vi "UHR-Fleezers Control (host) - 12.0.vi"() -> ()   [LabVIEW 2012] (continued)
            n680 = call "move to saved stage position.vi"("error in"=w1089, "Stage VISA resource name in"=w1090, "Position"="Stage Position To Establish FB", "Saved Stage Positions"=w1092) -> ("error out"=w1088:errorcluster)  [unwired: 1 out]
            n681 = local write "Stage Control Serial Error"(w1088) -> ()
          }
          frame #2 {
            n682 = call <vilib>:"Beep.vi"() -> ()  [unwired: 3 in, 9 out]
            n683 = Multiply(x="Wait (s)", y=u32 1000 ("milliseconds to wait")) -> (x*y=w1099:u32)
            n684 = property on="Trap Delta (MHz)" class="DigNum (strict)"("Val(Sgnl)"="Starting \nTrap Delta (MHz)") -> ()  [unwired: 2 in, 2 out]
            n685 = local write "Stage Moving"(FALSE ("Stage Moving")) -> ()
            n686 = Wait (ms)(milliseconds to wait=w1099) -> ()  [unwired: 1 out]
            n687 = property on="Tab Control 2" class="TabCtl (strict)"("Val(Sgnl)"=T6."Feedback on Trap Position" ("Value (Signaling)")) -> ()  [unwired: 2 in, 2 out]
            n688 = property on="Tab Control" class="TabCtl (strict)"("Val(Sgnl)"=T4."Trap Control (RF)" ("Value (Signaling)")) -> ()  [unwired: 2 in, 2 out]
          }
          frame #3 {
            n689 = property on="Set Reading to\nSetpoint" class="Bool (strict)"("Val(Sgnl)"=TRUE ("Value (Signaling)")) -> ()  [unwired: 2 in, 2 out]
            n690 = Wait (ms)(milliseconds to wait=u32 500) -> ()  [unwired: 1 out]
          }
          frame #4 {
            n691 = property on="Trap Pos. FB ON" class="Bool (strict)"("Val(Sgnl)"=TRUE ("Value (Signaling)")) -> ()  [unwired: 2 in, 2 out]
            n692 = Wait (ms)(milliseconds to wait=u32 250) -> ()  [unwired: 1 out]
          }
          frame #5 {
            n693 = case shown="False" "Trap Trig Fl." {
              frame False {
                n694 = case shown="True" "Green ON after FB ON?" {
                  selector: "Green ON after FB ON?" -> [_ w1114]
                  frame False {
                  }
                  frame True {
                    n695 = property on="Green Laser ON/Interlacing" class="Bool (strict)"("Val(Sgnl)"=w1114) -> ()  [unwired: 2 in, 2 out]
                  }
                }
              }
              frame True {
              }
            }
            n696 = case shown="True" "Remove Action Offset" {
              tunnel: TRUE ("Value (Signaling)") -> [w1111 w1112]
              frame False {
                n697 = property on="Remove Unwinding Offset" class="Bool (strict)"("Val(Sgnl)"=w1111) -> ()  [unwired: 2 in, 2 out]
              }
              frame True {
                n698 = property on="Remove Action Offset" class="Bool (strict)"("Val(Sgnl)"=w1112) -> ()  [unwired: 2 in, 2 out]
              }
            }
            n699 = Wait (ms)(milliseconds to wait=u32 250) -> ()  [unwired: 1 out]
          }
          frame #6 {
            n700 = property on="Start Saving" class="Bool (strict)"("Val(Sgnl)"=TRUE ("Value (Signaling)")) -> ()  [unwired: 2 in, 2 out]
            n701 = Wait (ms)(milliseconds to wait=u32 5000) -> ()  [unwired: 1 out]
          }
          frame #7 {
            w1118 = TRUE ("Value (Signaling)")
            n702 = property on="Rem fb disp offset" class="Bool (strict)"("Val(Sgnl)"=w1118) -> ()  [unwired: 2 in, 2 out]
            n703 = property on="Remove Offset" class="Bool (strict)"("Val(Sgnl)"=w1118) -> ()  [unwired: 2 in, 2 out]
            n704 = Wait (ms)(milliseconds to wait=u32 100) -> ()  [unwired: 1 out]
          }
          frame #8 {
            n705 = case shown="True" w1121 {
              frame False {
              }
              frame True {
                n706 = local write "Trap Trig. Fl."(TRUE ("Value (Signaling)")) -> ()
              }
            }
          }
          frame #9 {
            n707 = case shown="True" "Start dipping after?" {
              frame False {
              }
              frame True {
                n708 = flat-sequence {
                  frame #0 {
                    n709 = Multiply(x="Delay before dipping (s)", y=1000.0) -> (x*y=w1125:dbl)
                    n710 = Wait (ms)(milliseconds to wait=w1125) -> ()  [unwired: 1 out]
                  }
                  frame #1 {
                    n711 = property on="Dip for Protein" class="Bool (strict)"("Val(Sgnl)"=TRUE ("Value (Signaling)")) -> ()  [unwired: 2 in, 2 out]
                    n712 = local write "Scripts"(T1."Dipping" ("Scripts")) -> ()
                  }
                }
              }
            }
          }
        }
      }
      event "Fixed Traps Data\nScript": Value Change {
        n713 = event-data() -> ()  [unwired: 1 in, 5 out]
        n714 = flat-sequence {
          frame #0 {
            n715 = case shown="True" "Green ON" {
              frame False {
              }
              frame True {
                n716 = property on="Green Laser ON/Interlacing" class="Bool (strict)"("Val(Sgnl)"=TRUE) -> ()  [unwired: 2 in, 2 out]
              }
            }
            n717 = local write "Offset (nm)"(0.0 ("Offset (nm)")) -> ()
            n718 = property on="Sample Channel\nFlow" class="Bool (strict)"("Val(Sgnl)"=FALSE ("Value (Signaling)")) -> ()  [unwired: 2 in, 2 out]
            n719 = property on="Trap Delta (MHz)" class="DigNum (strict)"("Val(Sgnl)"="Fixed Traps Trap Delta (MHz)") -> ()  [unwired: 2 in, 2 out]
          }
          frame #1 {
            n720 = Wait (ms)(milliseconds to wait=u32 1000) -> ()  [unwired: 1 out]
          }
          frame #2 {
            n721 = local write "Start Saving"(TRUE ("Start Saving")) -> ()
          }
          frame #3 {
            n722 = local read "Bead Sep. Int. Time (s)"() -> (w1136:dbl)
            n723 = Multiply(x=w1136, y=1000.0) -> (x*y=w1138:dbl)
            n724 = Wait (ms)(milliseconds to wait=w1138) -> ()  [unwired: 1 out]
          }
          frame #4 {
            n725 = property on="Remove Offset" class="Bool (strict)"("Val(Sgnl)"=TRUE ("Value (Signaling)")) -> ()  [unwired: 2 in, 2 out]
          }
          frame #5 {
            n726 = property on="Dip for Protein" class="Bool (strict)"("Val(Sgnl)"="Start dipping after?") -> ()  [unwired: 2 in, 2 out]
          }
        }
      }
      event "Got DNA bead": Value Change {
        n727 = event-data() -> ()  [unwired: 1 in, 5 out]
        n728 = flat-sequence {
          frame #0 {
            n729 = local read "Daq spot flow on"() -> (w1143:bool)
            n730 = case shown="True" w1143 {
              frame False {
              }
              frame True {
                n731 = property on="Sample Channel\nFlow" class="Bool (strict)"("Val(Sgnl)"=TRUE ("Value (Signaling)")) -> ()  [unwired: 2 in, 2 out]
              }
            }
            n732 = property on="Got DNA bead" class="Bool"("Key Focus"=FALSE) -> ()  [unwired: 2 in, 2 out]
          }
          frame #1 {
            n733 = property on="Inject Pump 1" class="Bool (strict)"("Val(Sgnl)"=FALSE ("Value (Signaling)")) -> ()  [unwired: 2 in, 2 out]
          }
          frame #2 {
            n734 = property on="Cal/Data Acq. Spot" class="Bool (strict)"("Val(Sgnl)"=TRUE ("Value (Signaling)")) -> ()  [unwired: 2 in, 2 out]
          }
        }
      }
      event "Take Stepping Data": Value Change {
        n735 = event-data() -> ()  [unwired: 1 in, 5 out]
        n736 = local read "Save ave N"() -> (w1155:dbl)
        n737 = flat-sequence {
          tunnel: w1155 -> [w1157]
          tunnel: [w1157] -> w1150
          tunnel: [w1159] -> w1151
          tunnel: w1150 -> [w1159]
          tunnel: [w1161] -> w1152
          tunnel: w1151 -> [w1161]
          tunnel: [w1164] -> w1153
          tunnel: w1152 -> [w1164]
          tunnel: [w1166] -> w1154
          tunnel: w1153 -> [w1166]
          tunnel: [w1168] -> w1148
          tunnel: w1154 -> [w1168]
          tunnel: w1148 -> [w1171]
          tunnel: [w1171] -> w1147
          tunnel: w1147 -> [w1172]
          tunnel: [w1172] -> w1149
          tunnel: w1149 -> [w1178]
          frame #0 {
            n738 = property on="Save ave N" class="DigNum (strict)"("Val(Sgnl)"="Save ave factor") -> ()  [unwired: 2 in, 2 out]
          }
          frame #1 {
            n739 = Wait (ms)(milliseconds to wait=u32 100) -> ()  [unwired: 1 out]
          }
          frame #2 {
            n740 = local read "Offset 2 Start (MHz)"() -> (w1163:dbl)
            n741 = property on="Saved AOD Raster Scan Parameter Sets" class="Arr (strict)"("Index Values"=u32[] [2]) -> ()  [unwired: 2 in, 2 out]
            n742 = property on="Trap Delta (MHz)" class="DigNum (strict)"("Val(Sgnl)"=w1163) -> ()  [unwired: 2 in, 2 out]
          }
          frame #3 {
            n743 = property on="Load parameters" class="Bool (strict)"("Val(Sgnl)"=TRUE ("Value (Signaling)")) -> ()  [unwired: 2 in, 2 out]
          }
          frame #4 {
            n744 = Wait (ms)(milliseconds to wait=u32 100) -> ()  [unwired: 1 out]
          }
          frame #5 {
            n745 = property on="Trap Raster Scan" class="Bool (strict)"("Val(Sgnl)"=TRUE ("Value (Signaling)")) -> ()  [unwired: 2 in, 2 out]
          }
          frame #6 {
            n746 = Wait (ms)(milliseconds to wait=u32 1000) -> ()  [unwired: 1 out]
          }
          frame #7 {
            n747 = while {
              stop <- w1175 stop-if-true
              n748 = local read "Raster Scanning..."() -> (w1177:bool)
              n749 = local read "Saving..."() -> (w1176:bool)
              n750 = Not(x=w1176) -> (.not. x?=w1173:bool)
              n751 = Not(x=w1177) -> (.not. x?=w1174:bool)
              n752 = And(x=w1174, y=w1173) -> (x .and. y?=w1175:bool)
            }
          }
          frame #8 {
            n753 = property on="Save ave N" class="DigNum (strict)"("Val(Sgnl)"=w1178) -> ()  [unwired: 2 in, 2 out]
          }
        }
      }
      event "Step Size (nm)": Value Change {
        n754 = event-data() -> ()  [unwired: 1 in, 5 out]
        n755 = flat-sequence {
          frame #0 {
            n756 = property on="Saved AOD Raster Scan Parameter Sets" class="Arr (strict)"("Index Values"=u32[] [1]) -> ()  [unwired: 2 in, 2 out]
          }
          frame #1 {
            n757 = Multiply(x="N Steps", y="Step Size (nm)") -> (x*y=w1180:dbl)
            n758 = property on="Scan Speed AOD (nm/s) 2" class="DigNum (strict)"("Value"="Step Size (nm)") -> ()  [unwired: 2 in, 2 out]
            n759 = property on="Step Size AOD (nm) 2" class="DigNum (strict)"("Value"="Step Size (nm)") -> ()  [unwired: 2 in, 2 out]
            n760 = property on="Scan Range AOD (nm) 2" class="DigNum (strict)"("Value"=w1180) -> ()  [unwired: 2 in, 2 out]
          }
        }
      }
      event "Take Detection Laser\nImage": Value Change {
        n761 = event-data() -> ()  [unwired: 1 in, 5 out]
        n762 = flat-sequence {
          tunnel: [w1208] -> w1198
          tunnel: [w1207] -> w1191
          tunnel: [w1206] -> w1183
          tunnel: [w1211] -> w1199
          tunnel: w1198 -> [w1211]
          tunnel: [w1210] -> w1192
          tunnel: w1191 -> [w1210]
          tunnel: [w1209] -> w1184
          tunnel: w1183 -> [w1209]
          tunnel: [w1215] -> w1200
          tunnel: w1199 -> [w1215]
          tunnel: [w1214] -> w1193
          tunnel: w1192 -> [w1214]
          tunnel: [w1213] -> w1185
          tunnel: w1184 -> [w1213]
          tunnel: [w1221] -> w1201
          tunnel: w1200 -> [w1221]
          tunnel: [w1220] -> w1194
          tunnel: w1193 -> [w1220]
          tunnel: [w1219] -> w1186
          tunnel: w1185 -> [w1219]
          tunnel: [w1225] -> w1202
          tunnel: w1201 -> [w1225]
          tunnel: [w1224] -> w1195
          tunnel: w1194 -> [w1224]
          tunnel: [w1223] -> w1187
          tunnel: w1186 -> [w1223]
          tunnel: [w1229] -> w1203
          tunnel: w1202 -> [w1229]
          tunnel: [w1228] -> w1196
          tunnel: w1195 -> [w1228]
          tunnel: [w1227] -> w1188
          tunnel: w1187 -> [w1227]
          tunnel: [w1233] -> w1204
          tunnel: w1203 -> [w1233]
          tunnel: [w1232] -> w1197
          tunnel: w1196 -> [w1232]
          tunnel: [w1231] -> w1189
          tunnel: w1188 -> [w1231]
          tunnel: w1204 -> [w1239]
          tunnel: w1197 -> [w1238]
          tunnel: [w1236] -> w1190
          tunnel: w1189 -> [w1236]
          tunnel: w1190 -> [w1240]
          frame #0 {
            n763 = local read "Green Laser ON/Interlacing"() -> (w1208:bool)
            n764 = local read "Green laser mode"() -> (w1207:enum32{"Laser ON", "Laser OFF", "Interlace"})
            n765 = local read "Green FB On/Off"() -> (w1206:bool)
          }
          frame #1 {
            n766 = property on="Green FB On/Off" class="Bool (strict)"("Val(Sgnl)"=FALSE ("Value (Signaling)")) -> ()  [unwired: 2 in, 2 out]
          }
          frame #2 {
            n767 = property on="Green Laser ON/Interlacing" class="Bool (strict)"("Val(Sgnl)"=TRUE ("Value (Signaling)")) -> ()  [unwired: 2 in, 2 out]
            n768 = property on="Flip Green Filter" class="Bool (strict)"("Val(Sgnl)"=TRUE ("Value (Signaling)")) -> ()  [unwired: 2 in, 2 out]
            n769 = property on="Green laser mode" class="RadioBtnsControl (strict)"("Val(Sgnl)"=enum32{"Laser ON", "Laser OFF", "Interlace"}."Laser ON" ("Value (Signaling)")) -> ()  [unwired: 2 in, 2 out]
          }
          frame #3 {
            n770 = Wait (ms)(milliseconds to wait=u32 500) -> ()  [unwired: 1 out]
          }
          frame #4 {
            n771 = property on="Confocal Image" class="Bool (strict)"("Val(Sgnl)"=TRUE ("Value (Signaling)")) -> ()  [unwired: 2 in, 2 out]
          }
          frame #5 {
            n772 = Wait (ms)(milliseconds to wait=u32 2000) -> ()  [unwired: 1 out]
          }
          frame #6 {
            n773 = while {
              stop <- w1234 stop-if-true
              n774 = local read "Saving..."() -> (w1235:bool)
              n775 = Not(x=w1235) -> (.not. x?=w1234:bool)
            }
          }
          frame #7 {
            n776 = property on="Flip Green Filter" class="Bool (strict)"("Val(Sgnl)"=TRUE ("Value (Signaling)")) -> ()  [unwired: 2 in, 2 out]
            n777 = property on="Green Laser ON/Interlacing" class="Bool (strict)"("Val(Sgnl)"=w1239) -> ()  [unwired: 2 in, 2 out]
            n778 = property on="Green laser mode" class="RadioBtnsControl (strict)"("Val(Sgnl)"=w1238) -> ()  [unwired: 2 in, 2 out]
          }
          frame #8 {
            n779 = property on="Green FB On/Off" class="Bool (strict)"("Val(Sgnl)"=w1240) -> ()  [unwired: 2 in, 2 out]
          }
        }
      }
      event "Stop All": Value Change {
        n780 = event-data() -> ()  [unwired: 1 in, 5 out]
        n781 = local read "Stop All"() -> (w1241:bool)
      }
    }
    n782 = node-c288() -> ()  [unwired: 1 in, 1 out]
  }
  n783 = node-c288(3 ("Processor")) -> (w95:T21)  [unwired: 3 out]
  n784 = flat-sequence "Video" {
    tunnel: [w1251] -> w85
    tunnel: w85 -> [w1291]
    frame #0 {
      n785 = while {
        stop <- w1243 continue-if-true
        n786 = call "Close Video Capture.vi"() -> ("error code OUT"=w1245:i32)
        n787 = Equal?(x=w1245, y=0) -> (x = y?=w1243:bool)
      }
      n788 = local write "Stop All"(FALSE ("Stop All")) -> ()
    }
    frame #1 {
      n789 = call "DMR_Init.vi"() -> ()  [unwired: 3 out]
    }
    frame #2 {
      w1246 = "DE245428202"  # MSU fleezers card #
      (unwired) "DE019116701"  # Illinois fleezers card #
      # "Setting the destination format to Mono8 makes sure that the image can be displayed in the intensity plot."
      n790 = call "DMR_GetDevice.vi"("search string IN"=w1246) -> ("device handle OUT"=w1269:i32)  [unwired: 4 in, 2 out]
      n791 = call "DMR_OpenDevice.vi"("device handle IN"=w1269) -> ("driver handle OUT"=w1252:i32)  [unwired: 4 out]
      n792 = call "DMR_FindList.vi"("flags IN"=u32 0 ("flags"), "list name IN"="" ("String"), "list type IN"=T26."camera descriptions", "driver handle IN"=w1252) -> ("list handle OUT"=w1255:i32)  [unwired: 2 out]
      n793 = call "DMR_FindList.vi"("flags IN"=u32 0 ("flags"), "list name IN"="Base", "list type IN"=T26."setting", "driver handle IN"=w1252) -> ("list handle OUT"=w1253:i32)  [unwired: 2 out]
      n794 = call "OBJ_GetHandle.vi"("object name IN"="VideoStandard", "list handle IN"=w1255) -> ("object handle OUT"=w1249:i32)  [unwired: 3 out]
      n795 = call "OBJ_GetHandle.vi"("object name IN"="PixelFormat", "list handle IN"=w1253) -> ("object handle OUT"=w1263:i32)  [unwired: 3 out]
      n796 = call "OBJ_SetS.vi"("value index IN"=0, "value IN"="NTSC M", "object handle IN"=w1249) -> ()  [unwired: 2 out]
      n797 = call "OBJ_SetS.vi"("value index IN"=0, "value IN"="Mono8" ("value"), "object handle IN"=w1263) -> ()  [unwired: 2 out]
      n798 = call "OBJ_GetHandle.vi"("object name IN"="VideoChannel", "list handle IN"=w1253) -> ("object handle OUT"=w1259:i32)  [unwired: 3 out]
      n799 = while {
        tunnel: [w1273] -> w1251
        tunnel: w1252 -> [w1270]
        stop <- w1271 continue-if-true
        n800 = call "DMR_ImageRequestSingle.vi"("request control IN"=0, "driver handle IN"=w1270) -> ("error code OUT"=w1272:i32, "driver handle OUT"=w1273:i32)  [unwired: 2 out]
        n801 = Equal To 0?(x=w1272) -> (x = 0?=w1271:bool)
      }
      n802 = call "OBJ_SetI.vi"("value index IN"=0, "value IN"=3 ("Video channel"), "object handle IN"=w1259) -> ()  [unwired: 2 out]
    }
    frame #3 {
      w1279 = T17 0 items=["Grayscale (U8)", "Grayscale (I16)", "Grayscale (SGL)", "Complex (CSG)", "RGB (U32)", "HSL (U32)", "RGB (U64)"] ("Image Type")
      w1287 = T17 0 items=["Grayscale (U8)", "Grayscale (I16)", "Grayscale (SGL)", "Complex (CSG)", "RGB (U32)", "HSL (U32)", "RGB (U64)"] ("Image Type")
      n803 = for "Create Greyscale map" {
        N: 256 -> [_]
        tunnel: [w1293] -> w1276 mode=indexing
        workers-P: _ -> [_]
        i -> [w1296]
        n804 = To Unsigned Byte Integer(number=w1296) -> (unsigned 8bit integer=w1292:u8)
        n805 = Join Numbers(hi=w1292, lo=w1292) -> ((hi.lo)=w1295:u16)
        n806 = Join Numbers(hi=w1292, lo=w1292) -> ((hi.lo)=w1294:u16)
        n807 = Join Numbers(hi=w1295, lo=w1294) -> ((hi.lo)=w1293:u32)
      }
      n808 = call "IMAQ Create"("Image Name"="Scaled video", "Image Type"=w1279) -> ("New Image"=w1278:T2)  [unwired: 2 in, 2 out]
      n809 = call "IMAQ Create"("Image Name"="Main video", "Image Type"=w1287) -> ("New Image"=w1288:T2)  [unwired: 2 in, 2 out]
      n810 = node-c288(0 ("Processor")) -> (w1286:T21)  [unwired: 3 out]
      n811 = Initialize Array(u32 0 ("Window Number (0...15)"), 480 ("dimension size"), 640 ("dimension size")) -> (w1281:u32[][])
      n812 = timed-loop {
        tunnel: w1291 -> [w1313]
        tunnel: [w1312] -> w1290
        tunnel: w1288 -> [w1311]
        timing: w1286 -> [_]
        timing-out: [_] -> w1285
        tunnel: w1281 -> [w1300]
        tunnel: w1278 -> [w1298]
        tunnel: w1276 -> [w1297]
        stop <- w1299 stop-if-true
        # "This block performs the \nactual image capture."
        n813 = node-c288() -> ()  [unwired: 2 out]
        n814 = local read "Stop All"() -> (w1299:bool)
        n815 = Reciprocal(x="Video Capture Rate (Hz)") -> (1/x=w1303:dbl)
        n816 = Multiply(x=w1303, y=1000.0) -> (x*y=w1301:dbl)
        n817 = call "DMR_ImageRequestWaitFor.vi"("queue number IN"=0, "timeout(ms) IN"=500, "driver handle IN"=w1313) -> ("error code OUT"=w1317:i32, "request number OUT"=w1314:i32, "driver handle OUT"=w1315:i32)
        n818 = feedback #1(T27 refnum ("Avi Refnum")) -> (w1305:T27)
        n819 = case shown="True" "New Video File" {
          tunnel: [T27 refnum ("Avi Refnum") w1334] -> w1307
          tunnel: [FALSE TRUE] -> w1308
          tunnel: w1305 -> [_ w1330]
          frame False {
          }
          frame True {
            n820 = call "Create new save file.vi"("Ext"=".avi" ("string"), "Index In"="Video Index") -> ("Path Out"=w1326:path, "Index Out"=w1327:dbl)  [unwired: 1 in]
            "Path Out" <- w1326
            n821 = Not Equal?(x=w1330, y=T27 refnum ("Avi Refnum")) -> (x != y?=w1331:bool)
            n822 = Increment(x=w1327) -> (x+1=w1336:dbl)
            n823 = case shown="True" w1331 {
              tunnel: w1330 -> [_ w1337]
              frame False {
              }
              frame True {
                n824 = call "IMAQ AVI Close"("Avi Refnum"=w1337) -> ()  [unwired: 1 in, 10 out]
              }
            }
            n825 = local write "Video Index"(w1336) -> ()
            n826 = call "IMAQ AVI Create"("Frames Per Second"=u32 30, "AVI Path"=w1326) -> ("Avi Refnum"=w1334:T27)  [unwired: 5 in, 4 out]
          }
        }
        n827 = Equal To 0?(x=w1317) -> (x = 0?=w1316:bool)
        n828 = Select(t=w1307, s=w1308, f=w1305) -> (s? t:f=w1306:T27)
        n829 = feedback-in #1(w1306) -> ()
        n830 = case shown="True" w1316 {
          tunnel: w1315 -> [w1338 w1363]
          tunnel: w1314 -> [_ w1362]
          tunnel: [w1338 w1359] -> w1312
          tunnel: w1311 -> [_ w1343]
          tunnel: w1300 -> [_ w1347]
          tunnel: w1306 -> [_ w1345]
          tunnel: w1298 -> [_ w1340]
          tunnel: w1297 -> [_ w1339]
          frame False {
          }
          frame True {
            w1353 = u32 0 ("X-offset IN")
            n831 = call "DMR_GetImageRequestBufferData.vi"("driver handle IN"=w1363, "request number IN"=w1362) -> ("width OUT"=w1352:i32, "height OUT"=w1351:i32, "driver handle OUT"=w1358:i32, "request number OUT"=w1357:i32, "bytes per pixel OUT"=w1354:i32)  [unwired: 13 out]
            n832 = call "DMR_GetImageRequestBufferImageData.vi"("driver handle IN"=w1358, "request number IN"=w1357, "bytes per pixel IN"=w1354, "X-offset IN"=w1353, "Y-offset IN"=w1353, "height IN"=w1351, "width IN"=w1352) -> ("driver handle OUT"=w1356:u32, "request number OUT"=w1355:u32, "image OUT"=w1348:u32[][])  [unwired: 10 out]
            n833 = call "DMR_ImageRequestUnlock.vi"("request number IN"=w1355, "driver handle IN"=w1356) -> ("driver handle OUT"=w1361:i32)  [unwired: 1 in, 2 out]
            n834 = case shown="True" "Averaging" {
              tunnel: w1348 -> [w1399 w1404]
              tunnel: [w1399 w1403] -> w1344
              tunnel: w1347 -> [_ w1401]
              frame False {
              }
              frame True {
                (unwired) 1
                w1409 = 1
                n835 = feedback #2(w1401) -> (w1400:u32[][])
                n836 = Add(x=w1404, y=w1400) -> (x+y=w1405:u32[][])
                n837 = Select(t=w1401, s="Reset Averaging", f=w1405) -> (s? t:f=w1407:u32[][])
                n838 = feedback-in #2(w1407) -> ()
                n839 = feedback #3(w1409) -> (w1402:i32)
                n840 = Divide(x=w1405, y=w1402) -> (x/y=w1406:dbl[][])
                n841 = Increment(x=w1402) -> (x+1=w1410:i32)
                n842 = To Unsigned Long Integer(number=w1406) -> (unsigned 32bit integer=w1403:u32[][])
                n843 = Select(t=w1409, s="Reset Averaging", f=w1410) -> (s? t:f=w1408:i32)
                n844 = feedback-in #3(w1408) -> ()
              }
            }
            n845 = call "DMR_ImageRequestSingle.vi"("request control IN"=0, "driver handle IN"=w1361) -> ("driver handle OUT"=w1359:i32)  [unwired: 3 out]
            n846 = disable-structure shown="Disabled" {
              disable-tunnel: w1344 -> [w1376 _]
              disable-tunnel: w1340 -> [w1375 _]
              frame Disabled {
                n847 = To Double Precision Float(number=w1376) -> (double precision float=w1374:dbl[][])
                n848 = In Range and Coerce(upper limit="Intensity Upper", x=w1374, lower limit="Intensity Lower") -> (coerced(x)=w1373:dbl[][])  [unwired: 1 out]
                n849 = Subtract(x="Intensity Upper", y="Intensity Lower") -> (x-y=w1370:dbl)
                n850 = Subtract(x=w1373, y="Intensity Lower") -> (x-y=w1371:dbl[][])
                n851 = Divide(x=w1371, y=w1370) -> (x/y=w1372:dbl[][])
                n852 = Multiply(x=255.0, y=w1372) -> (x*y=w1368:dbl[][])
                n853 = To Unsigned Byte Integer(number=w1368) -> (unsigned 8bit integer=w1377:u8[][])
                n854 = call "IMAQ ArrayToImage"("Image Pixels (U8)"=w1377, "Image"=w1375) -> ("Image Out"=w1364:T2)  [unwired: 4 in, 5 out]
                n855 = First Call?() -> (First Call?: T/F=w1365:bool)
                n856 = case shown="True" w1365 {
                  tunnel: w1364 -> [w1378 w1389]
                  frame False {
                    n857 = flat-sequence {
                      tunnel: w1378 -> [w1384]
                      frame #0 {
                        w1381 = FALSE ("Get/Set Status? (Set)")
                        w1380 = 0 ("Window Number (0...15)")
                        n858 = call "IMAQ WindSize"("Get/Set Status? (Set)"=w1381, "Window Number"=w1380) -> ("Width & Height out"=→"Window Size":cluster{"Width":i32, "Height":i32})  [unwired: 4 in, 2 out]
                        n859 = call "IMAQ WindMove"("Window Number (0...15)"=w1380, "Get/Set Status? (Set)"=w1381) -> ("Coordinates (screen)"=→"Window Position":cluster{"X Position":i32, "Y Position":i32})  [unwired: 3 in, 1 out]
                        n860 = call "IMAQ WindDraw"("Resize to Image Size? (Y)"=FALSE, "Window Number (0...15)"=w1380, "Image"=w1384) -> ()  [unwired: 7 in, 2 out]
                      }
                      frame #1 {
                        n861 = call "IMAQ WindZoom 2"("Center Point"="Center Point", "Zoom to Fit? (False)"=FALSE, "Zoom Factor"="Zoom Factor") -> ()  [unwired: 5 in, 4 out]
                      }
                    }
                  }
                  frame True {
                    n862 = flat-sequence {
                      tunnel: w1389 -> [w1392]
                      tunnel: [w1390] -> w1388
                      tunnel: w1388 -> [w1394]
                      frame #0 {
                        w1391 = TRUE ("Resize to Image Size? (Y)")
                        w1390 = 0 ("Window Number (0...15)")
                        n863 = call "IMAQ WindNonTearing"("Window Number"=w1390, "NonTearing? (True)"=w1391) -> ()  [unwired: 8 in, 2 out]
                        n864 = call "IMAQ WindDraw"("Resize to Image Size? (Y)"=w1391, "Window Number (0...15)"=w1390, "Image"=w1392) -> ()  [unwired: 7 in, 2 out]
                      }
                      frame #1 {
                        n865 = call "IMAQ WindSize"("Scrollbars? (N)"=FALSE, "Width & Height"="Initial Window Size", "Window Number"=w1394) -> ()  [unwired: 3 in, 3 out]
                        n866 = call "IMAQ WindMove"("Window Number (0...15)"=w1394, "Coordinates (screen)"="Initial Window Position") -> ()  [unwired: 3 in, 2 out]
                      }
                    }
                  }
                }
              }
              frame Enabled {
              }
            }
            n867 = To Unsigned Byte Integer(number=w1344) -> (unsigned 8bit integer=w1342:u8[][])
            n868 = call "IMAQ ArrayToImage"("Image Pixels (U8)"=w1342, "Image"=w1343) -> ("Image Out"=w1341:T2)  [unwired: 4 in, 5 out]
            "Primary Video Display" <- w1341
            n869 = case shown="True" "Save Video" {
              tunnel: w1345 -> [_ w1398]
              tunnel: w1341 -> [_ w1397]
              frame False {
              }
              frame True {
                n870 = call "IMAQ AVI Write Frame"("Image"=w1397, "Avi Refnum"=w1398) -> ()  [unwired: 2 in, 8 out]
              }
            }
            n871 = case shown="True" "Save Image" {
              tunnel: w1342 -> [_ w1413]
              tunnel: w1339 -> [_ w1412]
              frame False {
              }
              frame True {
                n872 = call <vilib>:"Flatten Pixmap.vi"("colors"=w1412, "8-bit pixmap"=w1413) -> ("image data"=w1419:T28)  [unwired: 4 in, 5 out]
                n873 = call "Create new save file.vi"("Insert"="video_frame_" ("string"), "Ext"=".bmp" ("string"), "Index In"="Image Index") -> ("Path Out"=w1415:path, "Index Out"=w1420:dbl)
                n874 = Increment(x=w1420) -> (x+1=w1414:dbl)
                n875 = local write "Image Index"(w1414) -> ()
                n876 = call <vilib>:"Write BMP File.vi"("image data"=w1419, "path to BMP file"=w1415) -> ()  [unwired: 1 in, 9 out]
              }
            }
          }
        }
        n877 = node-c288(w1301) -> ()  [unwired: 1 out]
      }
      n878 = node-c288(w1285) -> ()  [unwired: 1 out]
      n879 = call "DMR_CloseDevice.vi"("driver handle IN"=w1290) -> ()  [unwired: 1 in, 4 out]
    }
    frame #4 {
      n880 = call "DMR_Close.vi"() -> ()  [unwired: 1 out]
    }
  }
  n881 = timed-loop "Acquire Data" {
    tunnel: w6 -> [w1712]
    tunnel: w55 -> [w1711]
    tunnel: [w1741] -> w274
    tunnel: [w1736] -> w272
    timing: w179 -> [_]
    timing-out: [_] -> w178
    tunnel: w74 -> [w1557]
    stop <- "Stop All" stop-if-true
    w1472 = "Initialize"
    w1542 = "NI_ChannelName" ("name")
    n882 = node-c288() -> ()  [unwired: 2 out]
    n883 = First Call?() -> (First Call?: T/F=w1507:bool)
    n884 = Or(x="Reset", y=w1507) -> (x .or. y?=w1508:bool)
    n885 = local read "Flushing P1"() -> (w1427:bool)
    n886 = case "Reset data stream" shown="True" w1508 {
      tunnel: w1712 -> [w2717 w2725]
      tunnel: w1711 -> [w2716 w2724]
      tunnel: [w2717 w2719] -> w1707
      tunnel: [w2716 w2718] -> w1706
      frame False {
      }
      frame True {
        w2722 = TRUE ("AI to FIFO")
        n887 = local write "Overflow (data lost)"(FALSE ("Overflow (data lost)")) -> ()
        n888 = call "reset FPGA DMA.vi"("error in"=w2724, "FPGA VI Reference In"=w2725) -> ("error out"=w2720:errorcluster, "FPGA VI Reference Out"=w2721:T19)
        n889 = xnode "Read/Write Control"("FPGA VI Reference In"=w2721, "error in"=w2720, "AI to FIFO"=w2722, "APD to FIFO"=w2722) -> ("FPGA VI Reference Out"=w2719:T19, "error out"=w2718:errorcluster)
      }
    }
    n890 = case shown="True" w1427 {
      frame False {
      }
      frame True {
        n891 = local read "Flush rate (uL/m) P1"() -> (w1758:dbl)
        n892 = local read "HP1 Flush Time (s)"() -> (w1767:dbl)
        n893 = local read "DMA Update Period (s)"() -> (w1761:dbl)
        n894 = Divide(x=w1758, y=60.0) -> (x/y=w1759:dbl)
        n895 = Divide(x=w1767, y=w1761) -> (x/y=w1756:dbl)
        n896 = feedback #4(0) -> (w1765:i32)
        n897 = Increment(x=w1765) -> (x+1=w1755:i32)
        n898 = Greater?(x=w1755, y=w1756) -> (0:w1764:bool)
        n899 = Compound Arithmetic op=MULTIPLY(w1761, w1755, w1759) -> (→"P1 Flush Volume (uL)":dbl)
        n900 = Divide(x=w1755, y=w1756) -> (x/y=→"P1 Flushing Bar":dbl)
        n901 = case shown="True" w1764 {
          tunnel: w1755 -> [w1768 _]
          tunnel: [w1768 0] -> w1763
          frame False {
          }
          frame True {
            w1769 = FALSE ("Flushing P1")
            n902 = local write "Inject Pump 1"(w1769) -> ()
            n903 = local write "Flushing P1"(w1769) -> ()
            n904 = property on="Clear Volume P1" class="Bool (strict)"("Val(Sgnl)"=TRUE ("Value (Signaling)")) -> ()  [unwired: 2 in, 2 out]
          }
        }
        n905 = feedback-in #4(w1763) -> ()
      }
    }
    n906 = Or(x="Start AOD Scan", y="Trap Raster Scan") -> (x .or. y?=w1663:bool)
    n907 = case "Start AOM raster scan" shown="True" w1663 {
      tunnel: w1707 -> [w2567 w2577]
      tunnel: w1706 -> [w2566 w2576]
      tunnel: [w2567 w2570] -> w1705
      tunnel: [w2566 w2569] -> w1704
      frame False {
      }
      frame True {
        n908 = case shown="True" "Restart DMA? (AOD)" {
          tunnel: [w2615 w2617] -> w2571
          tunnel: [w2614 w2616] -> w2572
          tunnel: w2577 -> [w2615 w2619]
          tunnel: w2576 -> [w2614 w2618]
          frame False {
          }
          frame True {
            n909 = local write "Overflow (data lost)"(FALSE ("Overflow (data lost)")) -> ()
            n910 = call "reset FPGA DMA.vi"("error in"=w2618, "FPGA VI Reference In"=w2619) -> ("error out"=w2616:errorcluster, "FPGA VI Reference Out"=w2617:T19)
          }
        }
        n911 = local write "Trap Raster Scan"(FALSE ("Trap Raster Scan")) -> ()
        n912 = case shown="True" "Move MCL Also?" {
          tunnel: w2572 -> [w2580 w2609]
          tunnel: w2571 -> [w2581 w2610]
          tunnel: [w2579 w2613] -> w2570
          tunnel: [w2578 w2612] -> w2569
          frame False {
            w2582 = TRUE ("AI to FIFO")
            n913 = xnode "Read/Write Control"("FPGA VI Reference In"=w2581, "error in"=w2580, "AI to FIFO"=w2582, "APD to FIFO"=w2582, "Start scan"=w2582) -> ("FPGA VI Reference Out"=w2579:T19, "error out"=w2578:errorcluster)
          }
          frame True {
            w2606 = FALSE ("1D or 2D Scan?")
            w2611 = TRUE ("AI to FIFO")
            # "Count for MCL loop"
            # "N total cycles"
            # "N steps"
            # "V_int"
            n914 = local read "Scan Range (nm)"() -> (w2588:dbl)
            n915 = local read "Number of F/B Scans (AOD)"() -> (w2605:u16)
            n916 = Sign(1:w2588) -> (0:w2587:dbl)
            n917 = Compound Arithmetic op=MULTIPLY(w2588, "MCL Step Position Ratio", "MCL/AOM Scale Tweak") -> (w2592:dbl)
            n918 = Negate(x=w2587) -> (-x=w2584:dbl)
            n919 = Multiply(x=w2584, y="MCL Step Increment (V_int)") -> (x*y=w2586:dbl)
            n920 = Divide(x=w2592, y="MCL X Cal (nm/V)") -> (x/y=w2598:dbl)
            n921 = Multiply(x=32767.0 ("y"), y=w2598) -> (x*y=w2604:dbl)
            n922 = local read "Total Counts (ticks)"() -> (w2589:u32)
            n923 = local read "Cycles/step (AOD)"() -> (w2600:u64)
            n924 = local read "Scan steps (AOD)"() -> (w2601:u64)
            n925 = Divide(x=w2604, y=10.0) -> (x/y=w2597:dbl)
            n926 = Divide(x=w2597, y="MCL Step Increment (V_int)") -> (x/y=w2595:dbl)
            n927 = Absolute Value(x=w2595) -> (abs(x)=w2583:dbl)
            n928 = Compound Arithmetic op=MULTIPLY(w2601, w2600, w2589) -> (w2596:u64)
            n929 = local write "wait to reset values"(w2611) -> ()
            n930 = local write "MCL Scanning"(w2611) -> ()
            n931 = Divide(x=w2596, y=w2583) -> (x/y=w2593:dbl)
            "MCL Count" <- w2593
            n932 = xnode "Read/Write Control"("FPGA VI Reference In"=w2610, "error in"=w2609, "Scan steps (MCL)"=w2583, "Number of scans (MCL)"=w2605, "Cycles per step (MCL)"=u64 1, "Scan freq.  increment (MCL)"=w2586, "1D or 2D Scan?"=w2606, "MCL Scan Axis"=w2606, "Cont. Scan (MCL)"=w2606, "MCL count"=w2593) -> ("FPGA VI Reference Out"=w2608:T19, "error out"=w2607:errorcluster)
            n933 = xnode "Read/Write Control"("FPGA VI Reference In"=w2608, "error in"=w2607, "AI to FIFO"=w2611, "APD to FIFO"=w2611, "Start scan"=w2611, "Start scan (MCL)"=w2611) -> ("FPGA VI Reference Out"=w2613:T19, "error out"=w2612:errorcluster)
          }
        }
        "Raster Scanning..." <- TRUE ("Scanning...")
      }
    }
    n934 = local read "Flushing P3"() -> (w1428:bool)
    n935 = case "Keep track of when Harvard Pump 3 is done flushing" shown="True" w1428 {
      frame False {
      }
      frame True {
        n936 = local read "Flush rate (uL/m) P3"() -> (w1775:dbl)
        n937 = local read "DMA Update Period (s)"() -> (w1777:dbl)
        n938 = local read "HP3 Flush Time (s)"() -> (w1784:dbl)
        n939 = Divide(x=w1775, y=60.0) -> (x/y=w1773:dbl)
        n940 = feedback #5(0) -> (w1782:i32)
        n941 = Increment(x=w1782) -> (x+1=w1776:i32)
        n942 = Divide(x=w1784, y=w1777) -> (x/y=w1778:dbl)
        n943 = Greater?(x=w1776, y=w1778) -> (0:w1781:bool)
        n944 = Compound Arithmetic op=MULTIPLY(w1777, w1776, w1773) -> (→"P3 Flush Volume (uL)":dbl)
        n945 = case shown="True" w1781 {
          tunnel: w1776 -> [w1785 _]
          tunnel: [w1785 0] -> w1780
          frame False {
          }
          frame True {
            w1786 = FALSE ("Flushing P3")
            n946 = local write "Inject Pump 3"(w1786) -> ()
            n947 = local write "Flushing P3"(w1786) -> ()
            n948 = property on="Clear Volume P3" class="Bool (strict)"("Val(Sgnl)"=TRUE ("Value (Signaling)")) -> ()  [unwired: 2 in, 2 out]
          }
        }
        n949 = feedback-in #5(w1780) -> ()
        n950 = Divide(x=w1776, y=w1778) -> (x/y=→"P3 Flushing Bar":dbl)
      }
    }
    n951 = And(x="Save scans", y=w1663) -> (x .and. y?=w1703:bool)
    n952 = Compound Arithmetic op=OR("Start MCL Scan", "Confocal Image", "Confocal Linescan") -> (w1661:bool)
    n953 = And(x="Save Data (MCL)", y=w1661) -> (x .and. y?=w1702:bool)
    n954 = case "Start MCL raster scan" shown="True" w1661 {
      tunnel: w1705 -> [w2184 w2200]
      tunnel: w1704 -> [w2183 w2199]
      tunnel: [w2184 w2195] -> w1555
      tunnel: [w2183 w2194] -> w1554
      tunnel: [FALSE w2193] -> w1688
      tunnel: "Start MCL Scan" -> [_ w2188]
      tunnel: "Confocal Image" -> [_ w2187]
      tunnel: "Confocal Linescan" -> [_ _]
      frame False {
      }
      frame True {
        w2193 = TRUE
        n955 = case shown="True" "Restart DMA? (MCL)" {
          tunnel: [w2245 w2247] -> w2198
          tunnel: [w2244 w2246] -> w2197
          tunnel: w2200 -> [w2245 w2250]
          tunnel: w2199 -> [w2244 w2249]
          frame False {
          }
          frame True {
            n956 = call "reset FPGA DMA.vi"("error in"=w2249, "FPGA VI Reference In"=w2250) -> ("error out"=w2246:errorcluster, "FPGA VI Reference Out"=w2247:T19)
            n957 = local write "Overflow (data lost)"(FALSE ("Overflow (data lost)")) -> ()
          }
        }
        n958 = case shown="False" w2188 {
          selector: w2188 -> [_ w2204]
          tunnel: w2187 -> [w2203 _]
          tunnel: [w2203 w2204] -> w2186
          frame False {
            n959 = property on="2D or 1D Scan" class="Bool (strict)"("Val(Sgnl)"=w2203) -> ()  [unwired: 2 in, 2 out]
            n960 = property on="Confocal Image" class="Bool (strict)"("Value"=FALSE ("Start Confocal Map")) -> ()  [unwired: 2 in, 2 out]
          }
          frame True {
          }
        }
        n961 = local write "MCL Scanning"(w2193) -> ()
        n962 = local read "AO1"() -> (w2190:dbl)
        n963 = local read "AO2"() -> (w2189:dbl)
        n964 = case shown="True" "Center Scan" {
          tunnel: w2198 -> [w2211 w2243]
          tunnel: w2197 -> [w2210 w2242]
          tunnel: [w2209 w2241] -> w2195
          tunnel: [w2208 w2240] -> w2194
          tunnel: [w2206 w2227] -> w2192
          tunnel: [w2205 w2226] -> w2191
          tunnel: w2190 -> [w2206 w2232]
          tunnel: w2189 -> [w2205 w2235]
          tunnel: w2186 -> [_ _]
          frame False {
            w2207 = TRUE ("AI to FIFO")
            n965 = xnode "Read/Write Control"("FPGA VI Reference In"=w2211, "error in"=w2210, "AI to FIFO"=w2207, "APD to FIFO"=w2207, "Start scan (MCL)"=w2207) -> ("FPGA VI Reference Out"=w2209:T19, "error out"=w2208:errorcluster)
          }
          frame True {
            w2239 = TRUE ("AI to FIFO")
            n966 = local read "Scan steps (MCL)"() -> (w2218:u64)
            n967 = local read "Scan lines (y)"() -> (w2214:u64)
            n968 = local read "Fast Scan Dir"() -> (w2225:bool)
            n969 = local read "Actual MCL Inc (V)"() -> (w2215:dbl)
            n970 = Decrement(x=w2214) -> (x-1=w2213:u64)
            n971 = Decrement(x=w2218) -> (x-1=w2217:u64)
            n972 = Multiply(x=w2215, y=w2213) -> (x*y=w2212:dbl)
            n973 = Divide(x=w2212, y=2.0) -> (x/y=w2222:dbl)
            n974 = Multiply(x=w2215, y=w2217) -> (x*y=w2216:dbl)
            n975 = Divide(x=w2216, y=2.0) -> (x/y=w2221:dbl)
            n976 = Select(t=w2221, s=w2225, f=w2222) -> (s? t:f=w2220:dbl)
            n977 = Select(t=w2222, s=w2225, f=w2221) -> (s? t:f=w2224:dbl)
            n978 = Subtract(x=w2232, y=w2224) -> (x-y=w2223:dbl)
            n979 = Subtract(x=w2235, y=w2220) -> (x-y=w2219:dbl)
            n980 = local read "2D or 1D Scan"() -> (w2237:bool)
            n981 = Not(x=w2225) -> (.not. x?=w2231:bool)
            n982 = Not(x=w2237) -> (.not. x?=w2233:bool)
            n983 = And(x=w2225, y=w2233) -> (x .and. y?=w2234:bool)
            n984 = And(x=w2233, y=w2231) -> (x .and. y?=w2236:bool)
            n985 = Select(t=w2235, s=w2236, f=w2219) -> (s? t:f=w2226:dbl)
            n986 = Select(t=w2232, s=w2234, f=w2223) -> (s? t:f=w2227:dbl)
            n987 = call "Volt to I16.vi"("Voltage In"=w2227) -> ("I16 Voltage Out"=w2230:i16)
            n988 = call "Volt to I16.vi"("Voltage In"=w2226) -> ("I16 Voltage Out"=w2229:i16)
            n989 = xnode "Read/Write Control"("FPGA VI Reference In"=w2243, "error in"=w2242, "AI to FIFO"=w2239, "APD to FIFO"=w2239, "Start scan (MCL)"=w2239, "AO1"=w2230, "AO2"=w2229) -> ("FPGA VI Reference Out"=w2241:T19, "error out"=w2240:errorcluster)
          }
        }
        "Initial Y" <- w2192
        "Initial X" <- w2191
        n990 = local write "Tab Control 6"(T3."Imaging" ("Tab Control 6")) -> ()
        "wait to reset values" <- w2193
      }
    }
    n991 = local read "Trap Pos Elements/DMA read"() -> (w1551:u32)
    n992 = local read "Trap AI Elements/DMA read"() -> (w1626:u32)
    n993 = local read "APD Elements/DMA read"() -> (w1592:u32)
    n994 = xnode "Get APD Data"("FPGA VI Reference In"=w1555, "error in"=w1554, "Number of Elements"=w1592, "Timeout (ms)"=-1) -> ("Data"=w1591:u32[], "Elements Remaining"=→"APD FIFO Elements Remaining":u32)  [unwired: 2 out]
    n995 = xnode "Invoke Method"("FPGA VI Reference In"=w1555, "error in"=w1554, "Number of Elements"=w1551, "Timeout (ms)"=-1) -> ("Data"=w1514:u16[], "Elements Remaining"=→"Trap Pos FIFO El Remaining":u32)  [unwired: 2 out]
    n996 = xnode "Get Trap Data"("FPGA VI Reference In"=w1555, "error in"=w1554, "Number of Elements"=w1626, "Timeout (ms)"=-1 ("Timeout")) -> ("FPGA VI Reference Out"=w1449:T19, "error out"=w1448:errorcluster, "Data"=w1515:i16[], "Elements Remaining"=w1749:u32)
    "FIFO El. Rem." <- w1749
    n997 = local read "Trap AI FIFO Depth"() -> (w1751:u32)
    n998 = Subtract(x=w1751, y=w1626) -> (x-y=w1750:u32)
    n999 = Decimate 1D Array(w1514) -> (w1511:u16[], w1513:u16[], w1512:u16[])
    n1000 = Divide(x=w1749, y=w1750) -> (x/y=w1748:dbl)
    "Buffer Status" <- w1748
    n1001 = To Unsigned Long Integer(number=w1511) -> (unsigned 32bit integer=w1510:u32[])
    n1002 = Join Numbers(hi=w1513, lo=w1512) -> ((hi.lo)=w1509:u32[])
    n1003 = Equal?(x=w1748, y=1.0) -> (x = y?=w1746:bool)
    n1004 = Join Numbers(hi=w1510, lo=w1509) -> ((hi.lo)=w1503:u64[])
    n1005 = call "IR AOM word to freq - vec.vi"("Frequency Word In (double vec)"=w1503) -> ("Frequency Out"=w1550:dbl[])
    n1006 = case "Alert buffer overflow" shown="True" w1746 {
      frame False {
      }
      frame True {
        n1007 = call <vilib>:"Beep.vi"() -> ()  [unwired: 3 in, 9 out]
        "Overflow (data lost)" <- TRUE ("Overflow (data lost)")
      }
    }
    n1008 = Decimate 1D Array(w1550) -> (w1549:dbl[], w1548:dbl[])
    n1009 = Build Array(w1549, w1548) -> (w1547:dbl[][])
    n1010 = local read "Trap Sets"() -> (w1625:u32)
    n1011 = case "Deinterlace trap data, average down PSD" shown="2" w1625 {
      tunnel: w1515 -> [w2280 w2345]
      tunnel: [w2277 w2342] -> w1618
      tunnel: [w2280 w2344] -> w1506
      tunnel: "Detector Type" -> [w2279 w2340]
      tunnel: [w2278 w2343] -> w1617
      tunnel: [w2276 w2341] -> w1723
      frame 1, Default {
        n1012 = Divide(x=w2280, y=3276.7) -> (x/y=w2281:dbl[])
        n1013 = Decimate 1D Array(w2281) -> (w2290:dbl[], w2289:dbl[], w2288:dbl[], w2287:dbl[], w2286:dbl[], w2285:dbl[], w2284:dbl[], w2283:dbl[])
        n1014 = case shown="\"IR-QPD + PSD + FB-QPD position\"" w2279 {
          tunnel: w2290 -> [w2314 w2339]
          tunnel: w2289 -> [w2313 w2338]
          tunnel: w2288 -> [w2298 w2316]
          tunnel: w2287 -> [w2299 w2326]
          tunnel: w2286 -> [w2312 w2337]
          tunnel: w2285 -> [w2311 w2336]
          tunnel: w2284 -> [w2295 w2317]
          tunnel: w2283 -> [w2294 w2315]
          tunnel: [w2293 w2323] -> w2278
          tunnel: [w2292 w2322] -> w2277
          tunnel: [w2291 w2321] -> w2276
          frame "IR-QPD + PSD + FB-QPD", Default {
            w2291 = 0  # Channel pattern
            n1015 = Divide(x=w2314, y=w2299) -> (x/y=w2301:dbl[])
            n1016 = Divide(x=w2313, y=w2299) -> (x/y=w2300:dbl[])
            n1017 = Divide(x=w2312, y=w2295) -> (x/y=w2297:dbl[])
            n1018 = Divide(x=w2311, y=w2294) -> (x/y=w2296:dbl[])
            n1019 = Build Array(w2301, w2300, w2299, w2298, w2297, w2296, w2295, w2294) -> (w2292:dbl[][])
            n1020 = Bundle("T1 Y", "T1 X", "T1 Sum", "FB Sum", "PSD Y", "PSD X", "PSD Y Sum", "PSD X Sum") -> (w2310:T37)  [unwired: 1 out]
            n1021 = Cluster To Array(cluster=w2310) -> (array=w2293:string[])
          }
          frame "IR-QPD + PSD + FB-QPD position" {
            w2321 = 3  # Channel pattern
            n1022 = Negate(x=w2317) -> (-x=w2318:dbl[])
            n1023 = Divide(x=w2339, y=w2326) -> (x/y=w2328:dbl[])
            n1024 = Divide(x=w2338, y=w2326) -> (x/y=w2327:dbl[])
            n1025 = Divide(x=w2337, y=w2317) -> (x/y=w2325:dbl[])
            n1026 = Divide(x=w2336, y=w2318) -> (x/y=w2324:dbl[])
            n1027 = Build Array(w2328, w2327, w2326, w2315, w2316, w2325, w2324, w2317) -> (w2322:dbl[][])
            n1028 = Bundle("T1 Y", "T1 X", "T1 Sum", "FB X", "FB Sum", "PSD Y", "PSD X", "PSD Y Sum") -> (w2335:T37)  [unwired: 1 out]
            n1029 = Cluster To Array(cluster=w2335) -> (array=w2323:string[])
          }
        }
      }
      frame 2 {
        n1030 = case shown="\"IR-QPD + PSD + FB-QPD X position\"" w2340 {
          tunnel: w2345 -> [w2407 w2474 w2545]
          tunnel: [w2346 w2465 w2476] -> w2344
          tunnel: [w2373 w2456 w2523] -> w2343
          tunnel: [w2372 w2419 w2490] -> w2342
          tunnel: [w2366 w2454 w2521] -> w2341
          frame "IR-QPD + PSD + FB-QPD", Default {
            w2366 = 1  # Channel pattern
            # "time average x2 the 4th signal and the 4 psd signals (detection laser)"
            # "deinterlace 3 signals from qpd"
            n1031 = Decimate 1D Array(w2407) -> (w2406:i16[], w2405:i16[], w2371:i16[], w2404:i16[], w2394:i16[], w2392:i16[], w2391:i16[], w2389:i16[])
            n1032 = Decimate 1D Array(w2371) -> (w2370:i16[], w2369:i16[])
            n1033 = Decimate 1D Array(w2406) -> (w2403:i16[], w2375:i16[])
            n1034 = Decimate 1D Array(w2405) -> (w2402:i16[], w2400:i16[])
            n1035 = Decimate 1D Array(w2404) -> (w2401:i16[], w2399:i16[])
            n1036 = call "downsample 1D array - double.vi"("Ave N"=2.0, "Array In"=w2394) -> ("Array Out"=w2393:dbl[])  [unwired: 1 out]
            n1037 = call "downsample 1D array - double.vi"("Ave N"=2.0, "Array In"=w2392) -> ("Array Out"=w2374:dbl[])  [unwired: 1 out]
            n1038 = call "downsample 1D array - double.vi"("Ave N"=2.0, "Array In"=w2391) -> ("Array Out"=w2390:dbl[])  [unwired: 1 out]
            n1039 = call "downsample 1D array - double.vi"("Ave N"=2.0, "Array In"=w2389) -> ("Array Out"=w2388:dbl[])  [unwired: 1 out]
            n1040 = Interleave 1D Arrays(w2403, w2402, w2401, w2375, w2400, w2399, w2370, w2369, w2393, w2374, w2390, w2388) -> (w2387:dbl[])
            n1041 = Divide(x=w2387, y=3276.7) -> (x/y=w2386:dbl[])
            n1042 = Decimate 1D Array(w2386) -> (w2385:dbl[], w2384:dbl[], w2383:dbl[], w2382:dbl[], w2381:dbl[], w2380:dbl[], w2368:dbl[], w2367:dbl[], w2379:dbl[], w2378:dbl[], w2377:dbl[], w2376:dbl[])
            n1043 = Divide(x=w2385, y=w2383) -> (x/y=w2353:dbl[])
            n1044 = Divide(x=w2384, y=w2383) -> (x/y=w2352:dbl[])
            n1045 = Divide(x=w2382, y=w2380) -> (x/y=w2351:dbl[])
            n1046 = Divide(x=w2381, y=w2380) -> (x/y=w2350:dbl[])
            n1047 = Divide(x=w2379, y=w2377) -> (x/y=w2349:dbl[])
            n1048 = Divide(x=w2378, y=w2376) -> (x/y=w2348:dbl[])
            n1049 = Build Array(w2353, w2352, w2383, w2351, w2350, w2380, w2368, w2367, w2349, w2348, w2377, w2376) -> (w2372:dbl[][])
            n1050 = Bundle("T1 Y", "T1 X", "T1 Sum", "T2 Y", "T2 X", "T2 Sum", "T1 FB Sum", "T2 FB Sum", "PSD Y", "PSD X", "PSD Y Sum", "PSD X Sum") -> (w2354:T38)  [unwired: 1 out]
            n1051 = To Word Integer(number=w2387) -> (16bit integer=w2346:i16[])
            n1052 = Cluster To Array(cluster=w2354) -> (array=w2373:string[])
          }
          frame "IR-QPD + PSD + FB-QPD X position" {
            w2454 = 2  # Channel pattern
            # "time average x2 the 3 psd signals (detection laser)"
            # "deinterlace 3 signals from qpds"
            n1053 = Decimate 1D Array(w2474) -> (w2473:i16[], w2472:i16[], w2455:i16[], w2471:i16[], w2417:i16[], w2414:i16[], w2411:i16[], w2442:i16[])
            n1054 = Decimate 1D Array(w2455) -> (w2440:i16[], w2438:i16[])
            n1055 = Decimate 1D Array(w2473) -> (w2470:i16[], w2457:i16[])
            n1056 = Decimate 1D Array(w2472) -> (w2469:i16[], w2467:i16[])
            n1057 = Decimate 1D Array(w2471) -> (w2468:i16[], w2466:i16[])
            n1058 = Decimate 1D Array(w2442) -> (w2441:i16[], w2439:i16[])
            n1059 = call "downsample 1D array - I16.vi"("Ave N"=2.0, "Array In"=w2417) -> ("Array Out"=w2415:i16[])  [unwired: 1 in]
            n1060 = call "downsample 1D array - I16.vi"("Ave N"=2.0, "Array In"=w2411) -> ("Array Out"=w2409:i16[])  [unwired: 1 in]
            n1061 = call "downsample 1D array - I16.vi"("Ave N"=2.0, "Array In"=w2414) -> ("Array Out"=w2412:i16[])  [unwired: 1 in]
            n1062 = Interleave 1D Arrays(w2470, w2469, w2468, w2457, w2467, w2466, w2441, w2440, w2439, w2438, w2415, w2412, w2409) -> (w2465:i16[])
            n1063 = Divide(x=w2465, y=3276.7) -> (x/y=w2464:dbl[])
            n1064 = Decimate 1D Array(w2464) -> (w2463:dbl[], w2462:dbl[], w2461:dbl[], w2460:dbl[], w2459:dbl[], w2458:dbl[], w2430:dbl[], w2428:dbl[], w2427:dbl[], w2425:dbl[], w2424:dbl[], w2423:dbl[], w2420:dbl[])
            n1065 = Negate(x=w2420) -> (-x=w2418:dbl[])
            n1066 = Divide(x=w2424, y=w2420) -> (x/y=w2422:dbl[])
            n1067 = Divide(x=w2423, y=w2418) -> (x/y=w2421:dbl[])
            n1068 = Divide(x=w2463, y=w2461) -> (x/y=w2446:dbl[])
            n1069 = Divide(x=w2462, y=w2461) -> (x/y=w2445:dbl[])
            n1070 = Divide(x=w2460, y=w2458) -> (x/y=w2444:dbl[])
            n1071 = Divide(x=w2459, y=w2458) -> (x/y=w2443:dbl[])
            n1072 = Divide(x=w2430, y=w2428) -> (x/y=w2429:dbl[])
            n1073 = Divide(x=w2427, y=w2425) -> (x/y=w2426:dbl[])
            n1074 = Build Array(w2446, w2445, w2461, w2444, w2443, w2458, w2429, w2428, w2426, w2425, w2422, w2421, w2420) -> (w2419:dbl[][])
            n1075 = Bundle("T1 Y", "T1 X", "T1 Sum", "T2 Y", "T2 X", "T2 Sum", "T1 FB X", "T1 FB Sum", "T2 FB X", "T2 FB Sum", "PSD Y", "PSD X", "PSD Y Sum") -> (w2447:T39)  [unwired: 1 out]
            n1076 = Cluster To Array(cluster=w2447) -> (array=w2456:string[])
          }
          frame "IR-QPD + PSD + FB-QPD XY positions" {
            w2521 = 4  # Channel pattern
            # "time average x2 the 3 psd signals (detection laser)"
            # "deinterlace 3 signals from qpds"
            n1077 = Decimate 1D Array(w2545) -> (w2544:i16[], w2543:i16[], w2522:i16[], w2542:i16[], w2488:i16[], w2534:i16[], w2533:i16[], w2510:i16[])
            n1078 = Decimate 1D Array "Feedback Sum"(w2522) -> (w2506:i16[], w2504:i16[])
            n1079 = Decimate 1D Array "QPD Y"(w2544) -> (w2541:i16[], w2524:i16[])
            n1080 = Decimate 1D Array "QPD X"(w2543) -> (w2540:i16[], w2538:i16[])
            n1081 = Decimate 1D Array "Feedback Y"(w2488) -> (w2487:i16[], w2486:i16[])
            n1082 = Decimate 1D Array "QPD Sum"(w2542) -> (w2539:i16[], w2537:i16[])
            n1083 = Decimate 1D Array "Feedback X"(w2510) -> (w2507:i16[], w2505:i16[])
            n1084 = call "downsample 1D array - double.vi"("Ave N"=2.0, "Array In"=w2534) -> ("Array Out"=w2509:dbl[])  [unwired: 1 out]
            n1085 = call "downsample 1D array - double.vi"("Ave N"=2.0, "Array In"=w2533) -> ("Array Out"=w2508:dbl[])  [unwired: 1 out]
            n1086 = Interleave 1D Arrays(w2541, w2540, w2539, w2524, w2538, w2537, w2487, w2507, w2506, w2486, w2505, w2504, w2509, w2508) -> (w2532:dbl[])
            n1087 = Divide(x=w2532, y=3276.7) -> (x/y=w2531:dbl[])
            n1088 = Decimate 1D Array(w2531) -> (w2530:dbl[], w2529:dbl[], w2528:dbl[], w2527:dbl[], w2526:dbl[], w2525:dbl[], w2483:dbl[], w2497:dbl[], w2481:dbl[], w2482:dbl[], w2495:dbl[], w2479:dbl[], w2493:dbl[], w2491:dbl[])
            n1089 = Negate(x=w2491) -> (-x=w2489:dbl[])
            n1090 = Divide(x=w2493, y=w2489) -> (x/y=w2492:dbl[])
            n1091 = Divide(x=w2482, y=w2479) -> (x/y=w2478:dbl[])
            n1092 = Divide(x=w2483, y=w2481) -> (x/y=w2480:dbl[])
            n1093 = Divide(x=w2530, y=w2528) -> (x/y=w2514:dbl[])
            n1094 = Divide(x=w2529, y=w2528) -> (x/y=w2513:dbl[])
            n1095 = Divide(x=w2527, y=w2525) -> (x/y=w2512:dbl[])
